vi "Apply.vi"(8 "error in (no error)":errorcluster, 11 "DAQmx Base CFG in":refnum<class "DAQmx Base CFG.lvclass">) -> (0 "error out":errorcluster, 3 "DAQmx Base CFG out":refnum<class "DAQmx Base CFG.lvclass">)   [LabVIEW 2023, in "DAQmx Base CFG.lvclass"]
uses:
  DAQmx Base CFG.lvclass
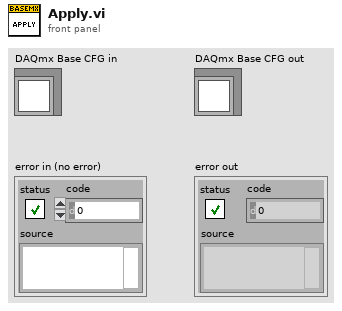
[diagram p1: front panel]
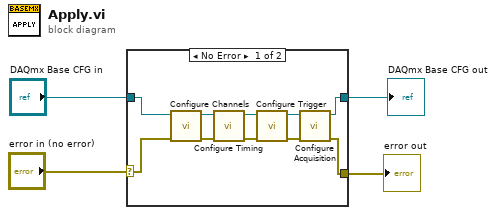
[diagram p0: block diagram]
diagram:
  n1 = case shown="No Error" "error in (no error)" {
    selector: "error in (no error)" -> [w13 w16]
    tunnel: "DAQmx Base CFG in" -> [w14 w15]
    tunnel: [w12 w16] -> w2
    tunnel: [w11 w15] -> w1
    frame No Error {
      n2 = call-dynamic "Configure Channels.vi"("error in (no error)"=w13, "DAQmx Base CFG in"=w14) -> ("error out"=w9:errorcluster, "DAQmx Base CFG out"=w10:refnum<class "DAQmx Base CFG.lvclass">)  [unwired: 8 in]
      n3 = call-dynamic "Configure Timing.vi"("error in (no error)"=w9, "DAQmx Base CFG in"=w10) -> ("error out"=w7:errorcluster, "DAQmx Base CFG out"=w8:refnum<class "DAQmx Base CFG.lvclass">)  [unwired: 8 in]
      n4 = call-dynamic "Configure Trigger.vi"("error in (no error)"=w7, "DAQmx Base CFG in"=w8) -> ("error out"=w5:errorcluster, "DAQmx Base CFG out"=w6:refnum<class "DAQmx Base CFG.lvclass">)  [unwired: 8 in]
      n5 = call-dynamic "Configure Acquisition.vi"("error in (no error)"=w5, "DAQmx Base CFG in"=w6) -> ("error out"=w12:errorcluster, "DAQmx Base CFG out"=w11:refnum<class "DAQmx Base CFG.lvclass">)  [unwired: 8 in]
    }
    frame Error {
    }
  }
  "error out" <- w2
  "DAQmx Base CFG out" <- w1
